vi "compilerUpdate.vi"(6 "String":string="    Compiler Error", 8 "error in (no error)":errorcluster, 9 "Path":path, 10 "Listbox in":refnum<vi>, 11 "ExperimentRunner in":refnum<class "ExperimentRunner.lvclass">) -> (0 "error out":errorcluster, 2 "Listbox out":refnum<vi>, 3 "ExperimentRunner out":refnum<class "ExperimentRunner.lvclass">)   [LabVIEW 2011, in "Views.lvlib" / "ExperimentControl.lvlib" / "ExperimentRunner.lvclass"]
uses:
  ExperimentRunner.lvclass
  ExperimentRunner.lvclass/ExperimentRunner.ctl
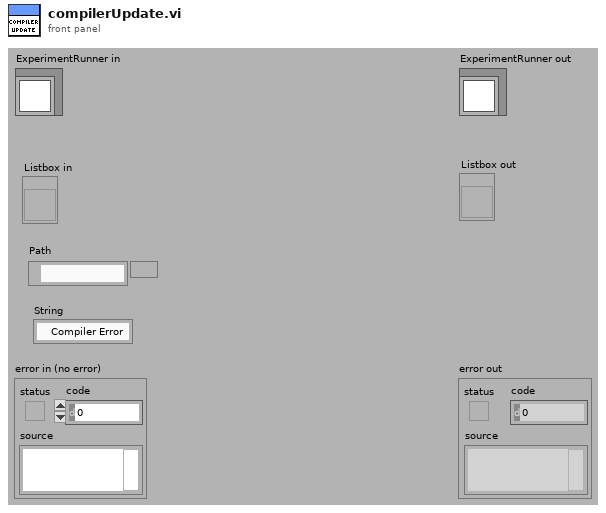
[diagram p1: front panel]
types:
  T1 = cluster{"CompilerPath":path, "CompilerString":string}[]
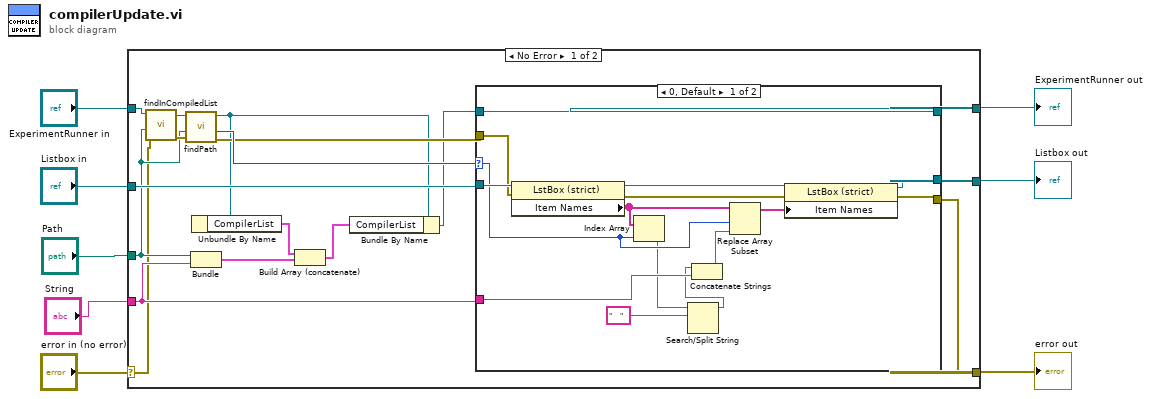
[diagram p0: block diagram]
diagram:
  n1 = case shown="No Error" "error in (no error)" {
    selector: "error in (no error)" -> [w9 w46]
    tunnel: [w20 w46] -> w7
    tunnel: [w22 w45] -> w5
    tunnel: "ExperimentRunner in" -> [w11 w45]
    tunnel: "Path" -> [w10 _]
    tunnel: "Listbox in" -> [w23 w44]
    tunnel: [w21 w44] -> w2
    tunnel: "String" -> [w17 _]
    frame No Error {
      n2 = call "findInCompiledList.vi"("error in (no error)"=w9, "Path"=w10, "ExperimentRunner in"=w11) -> ("error out"=w12:errorcluster, "ExperimentRunner out"=w13:refnum<class "ExperimentRunner.lvclass">)  [unwired: 7 in]
      n3 = call "findPath.vi"("error in (no error)"=w12, "Path"=w10, "ExperimentRunner in"=w13) -> ("error out"=w24:errorcluster, "index of element"=w25:i32, "ExperimentRunner out"=w18:refnum<class "ExperimentRunner.lvclass">)  [unwired: 6 in]
      n4 = Bundle("Path"=w10, "String"=w17) -> (w14:cluster{"Path":path, "String":string})  [unwired: 1 in]
      n5 = Unbundle By Name(w18) -> ("CompilerList"=w16:T1)
      n6 = Build Array (concatenate)(w16, w14) -> (w15:cluster{"Path":path, "String":string}[])
      n7 = Bundle By Name(cluster=w18, "CompilerList"=w15) -> (w19:refnum<class "ExperimentRunner.lvclass">)
      n8 = case shown="0, Default" w25 {
        selector: w25 -> [w35 _]
        tunnel: w19 -> [w40 w43]
        tunnel: w24 -> [w38 w41]
        tunnel: w23 -> [w39 w42]
        tunnel: [w40 w43] -> w22
        tunnel: [w31 w42] -> w21
        tunnel: [w30 w41] -> w20
        tunnel: w17 -> [w29 _]
        frame 0, Default {
          n9 = property class="LstBox (strict)"(reference=w39, error in=w38) -> (reference out=w34:refnum<vi>, error out=w33:errorcluster, "Item Names"=w36:string[])
          n10 = Index Array(array=w36, index=w35) -> (element=w27:string)
          n11 = Search/Split String(string=w27, search string/char (-)="    ") -> (substring before match=w28:string)  [unwired: 1 in, 2 out]
          n12 = Concatenate Strings(w28, w29) -> (w37:string)
          n13 = Replace Array Subset(array=w36, new element=w37, index=w35) -> (w32:string[])
          n14 = property class="LstBox (strict)"(reference=w34, error in=w33, "Item Names"=w32) -> (reference out=w31:refnum<vi>, error out=w30:errorcluster)
        }
        frame -1 {
        }
      }
    }
    frame Error {
    }
  }
  "error out" <- w7
  "ExperimentRunner out" <- w5
  "Listbox out" <- w2
